vi "Write Arguments.vi"(8 "error in (no error)":errorcluster, 10 "Arguments":variant, 11 "Command in":refnum<class "Command.lvclass">) -> (0 "error out":errorcluster, 3 "Command out":refnum<class "Command.lvclass">)   [LabVIEW 2017, in "Message Interface.lvlib" / "Command.lvclass"]
uses:
  Command.lvclass
  Command.lvclass/Command.ctl
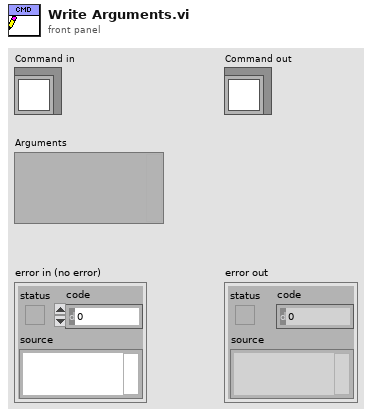
[diagram p1: front panel]
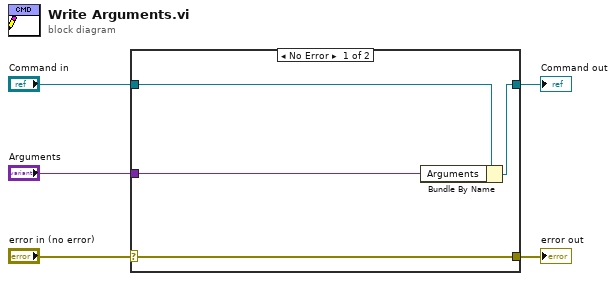
[diagram p0: block diagram]
diagram:
  n1 = case shown="No Error" "error in (no error)" {
    selector: "error in (no error)" -> [w9 w10]
    tunnel: [w9 w10] -> w4
    tunnel: [w7 w11] -> w2
    tunnel: "Command in" -> [w8 w11]
    tunnel: "Arguments" -> [w6 _]
    frame No Error {
      n2 = Bundle By Name(cluster=w8, "Arguments"=w6) -> (w7:refnum<class "Command.lvclass">)
    }
    frame Error {
    }
  }
  "error out" <- w4
  "Command out" <- w2
